vi "CRC16CITT.vi"   [LabVIEW 2019]
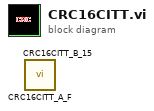
[diagram p0: block diagram]
diagram:
  n1 = call "CRC16CITT_A_F.vi"() -> ()  [unwired: 9 in, 3 out]
  n2 = call "CRC16CITT_B_15.vi"() -> ()  [unwired: 9 in, 3 out]
